vi "sim_scope_2.vi"(7 "CHAN":T1={"channel name"="CHANNEL2", "probe attenuation"=1.0, "vertical offset"=0.0, "vertical range"=1.0, "vertical coupling"=1, "input impedance"=50.0} {"input impedance" format="%#_13g"; "vertical coupling" items=["AC", "DC", "GND"]; "vertical range" format="%.3f"; "vertical offset" format="%.3f"; "probe attenuation" format="%.3f"}, 9 "noise":dbl=0.1 format="%#_13g", 10 "dt":dbl=1e-08 format="%#_2e", 11 "Points":i32=1000) -> (2 "output waveform":waveform(dbl)={"t0"=timestamp(0 s since 1904-01-01), "dt"=1e-08, "Y"=array[1000 elements]})   [LabVIEW 2015, in "daq_simulate.lvlib"]
uses:
  daq_simulate.lvlib
  fake_oscilloscope/osc_channel.ctl
panel:
  in  "A":dbl=1.0 format="%#_13g"
  in  "eff":dbl=0.25
  in  "tau":dbl=1.42e-07
  in  "sigma":dbl=1e-08
  out "min":dbl=-0.5
  out "max":dbl=0.5
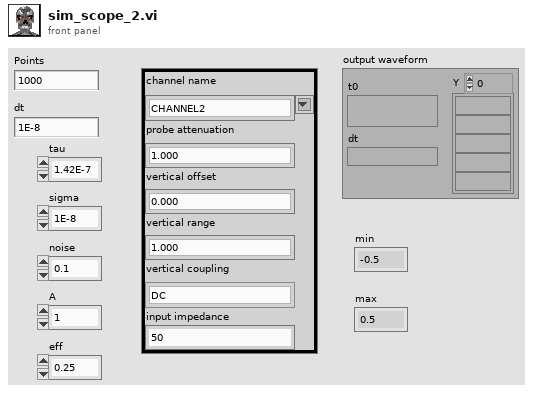
[diagram p1: front panel]
types:
  T1 = typedef "osc_channel.ctl" = cluster{"channel name":string, "probe attenuation":dbl, "vertical offset":dbl, "vertical range":dbl, "vertical coupling":i32, "input impedance":dbl}
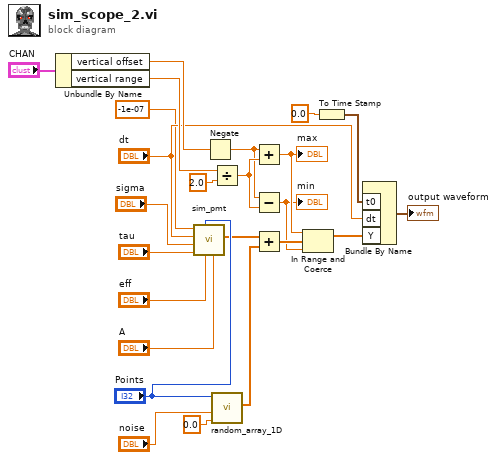
[diagram p0: block diagram]
diagram:
  n1 = Unbundle By Name("CHAN") -> ("vertical offset"=w13:dbl, "vertical range"=w16:dbl)
  n2 = call "sim_pmt.vi"("A"="A", "eff"="eff", "N"="Points", "tau"="tau", "sigma"="sigma", "dx"="dt", "x0"=-1e-07) -> ("y"=w2:dbl[])  [unwired: 3 in, 1 out]
  n3 = Negate(x=w13) -> (-x=w12:dbl)
  n4 = Divide(x=w16, y=2.0) -> (x/y=w14:dbl)
  n5 = call "random_array_1D.vi"("offset"=0.0, "scale"="noise", "N"="Points") -> ("Array"=w23:dbl[])  [unwired: 8 in]
  n6 = Add(x=w12, y=w14) -> (x+y=w11:dbl)
  "max" <- w11
  n7 = Subtract(x=w12, y=w14) -> (x-y=w10:dbl)
  "min" <- w10
  n8 = Add(x=w2, y=w23) -> (x+y=w19:dbl[])
  n9 = In Range and Coerce(upper limit=w11, x=w19, lower limit=w10) -> (coerced(x)=w18:dbl[])  [unwired: 1 out]
  n10 = To Time Stamp(1:0.0 ("number")) -> (0:w24:timestamp)
  n11 = Bundle By Name("t0"=w24, "dt"="dt", "Y"=w18) -> (→"output waveform":waveform(dbl))  [unwired: 1 in]
